vi "Insert into tabella db.vi"(8 "error in (no error)":errorcluster, 9 "Array":string[](array[string]), 10 "table":string, 11 "Refnum in":T1) -> (0 "error out":errorcluster, 3 "connection reference":T1)   [LabVIEW 2014]
uses:
  <vilib>/addons/database/Connection.llb/Conn ObjectReference.ctl
  <vilib>/addons/database/Connection.llb/Conn Execute.vi
  <vilib>/addons/database/Recordset.llb/Rec Destroy - Connection.vi
  <vilib>/addons/database/NI_Database_API.lvlib
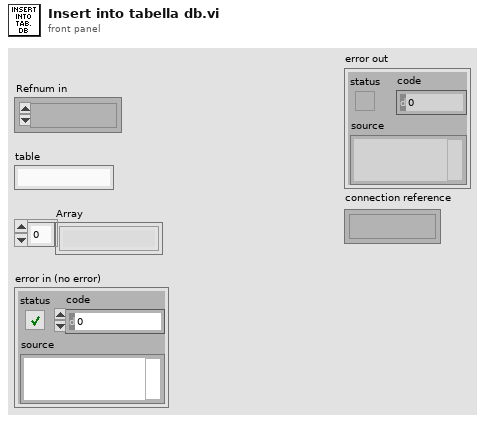
[diagram p1: front panel]
types:
  T1 = typedef "NI_Database_API.lvlib/Conn ObjectReference.ctl" = refnum<k1>
  T2 = typedef "NI_Database_API.lvlib/Rec ObjectReference.ctl" = refnum<k1>
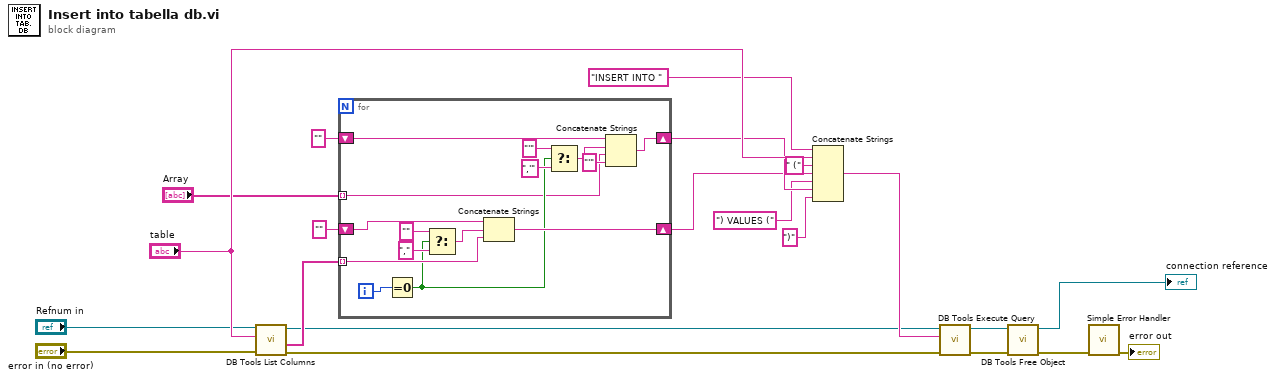
[diagram p0: block diagram]
diagram:
  n1 = call <vilib>:"DB Tools List Columns.vi"("error in (no error)"="error in (no error)", "table"="table", "connection reference"="Refnum in") -> ("error out"=w9:errorcluster, "columns"=w10:string[], "connection reference out"=w8:T1)  [unwired: 1 in, 1 out]
  n2 = for {
    tunnel: w10 -> [w32] mode=indexing
    shift-right: [w31] -> w12
    shift-left: "" -> [w36]
    shift-right: [w23] -> w15
    shift-left: "" -> [w26]
    tunnel: "Array" -> [w22] mode=indexing
    i -> [w24]
    n3 = Equal To 0?(x=w24) -> (x = 0?=w27:bool)
    n4 = Select(t="", s=w27, f=",") -> (s? t:f=w33:string)
    n5 = Concatenate Strings(w36, w33, w32) -> (w31:string)
    n6 = Select(t="'", s=w27, f=",'") -> (s? t:f=w30:string)
    n7 = Concatenate Strings(w26, w30, w22, "'" ("string")) -> (w23:string)
  }
  n8 = Concatenate Strings("INSERT INTO " ("SQL query"), "table", " (" ("string"), w12, ") VALUES (" ("string"), w15, ")" ("string")) -> (w17:string)
  n9 = call-poly <vilib>:"DB Tools Execute Query.vi"("error in (no error)"=w9, "SQL query"=w17, "connection reference"=w8) -> ("error out"=w4:errorcluster, "recordset reference"=w2:T2)  [unwired: 5 in]
  n10 = call-poly <vilib>:"DB Tools Free Object.vi"("error in (no error)"=w4, "recordset reference"=w2) -> ("error out"=w3:errorcluster, "connection reference"=→"connection reference":T1)  [unwired: 8 in]
  n11 = call <vilib>:"Simple Error Handler.vi"("error in (no error)"=w3) -> ("error out"=→"error out":errorcluster)  [unwired: 4 in, 4 out]
